vi "Driver - DTACQ - Flush Read Buffer.vi"(8 "error in":errorcluster, 11 "DTACQ Connection Data In":T1={"Description"="", "Address"="", "Port"=0, "timeout (ms)"=5000, "Termination Character"="\n", "TCP Connection Reference"=refnum, "Open Connection"=FALSE}) -> (0 "error out":errorcluster, 3 "DTACQ Connection Data Out":T1={"Description"="", "Address"="", "Port"=0, "timeout (ms)"=5000, "Termination Character"="\n", "TCP Connection Reference"=refnum, "Open Connection"=FALSE})   [LabVIEW 2017, in "Communications Library.lvlib"]
doc: "Clears any characters in the read buffer."
uses:
  Communications Library.lvlib
  Typedefs/DTACQ Connection Data--Cluster.ctl
  <vilib>/Utility/error.llb/Clear Errors.vi
  Debug - Lower Level - Logging Tool.vi
  Error 5102 - DTACQ unit replied with an error--const.vi
  Debug - TCP - Write to Log File.vi
  Debug - TCP - Create Descriptive String.vi
  <vilib>/Utility/error.llb/Error Cluster From Error Code.vi
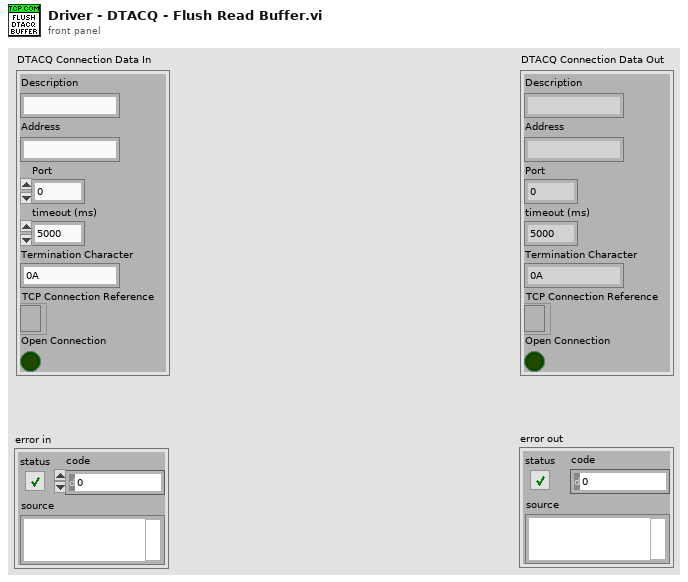
[diagram p1: front panel]
types:
  T1 = typedef "Communications Library.lvlib/DTACQ Connection Data--Cluster.ctl" = cluster{"Description":string, "Address":string, "Port":u16, "timeout (ms)":i32, "Termination Character":string, "TCP Connection Reference":refnum<k5>, "Open Connection":bool}
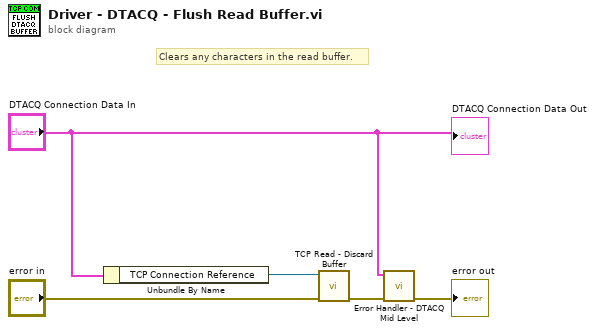
[diagram p0: block diagram]
diagram:
  # "Clears any characters in the read buffer."
  n1 = Unbundle By Name("DTACQ Connection Data In") -> ("TCP Connection Reference"=w5:refnum<k5>)
  n2 = call "TCP Read - Discard Buffer.vi"("error in"="error in", "TCP Network Connection in"=w5) -> ("error out"=w3:errorcluster)  [unwired: 7 in, 2 out]
  n3 = call "Error Handler - DTACQ Mid Level.vi"("error in"=w3, "DTACQ Connection Data In"="DTACQ Connection Data In") -> ("error out"=→"error out":errorcluster)  [unwired: 7 in, 2 out]
  "DTACQ Connection Data Out" <- "DTACQ Connection Data In"
